vi "ObservedPVs.vi"(8 "error in":errorcluster[](array[cluster]), 10 "Observed PVs":cluster{"PV-Name":string, "n-Channels?":bool}[](array[cluster])=[{"PV-Name"="Waveform", "n-Channels?"=FALSE}, {"PV-Name"="VerticalRange", "n-Channels?"=TRUE}], 11 "PVs":T1(array[cluster])) -> (0 "error out":errorcluster[](array[cluster]), 3 "PVs":T1(array[cluster]))   [LabVIEW 2015, in "CS++ScopeGui.lvlib" / "CS++ScopeGui.lvclass"]
uses:
  CS++ScopeGui.lvclass
  CSPP_Core/Actors/CS++GUIActor Messages/Update-PV Msg/Update-PV Msg.lvclass
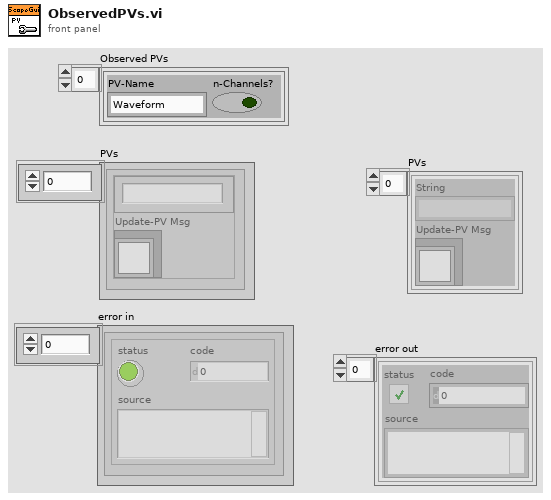
[diagram p1: front panel]
types:
  T1 = cluster{"String":string, "Update-PV Msg":refnum<class "Update-PV Msg.lvclass">}[]
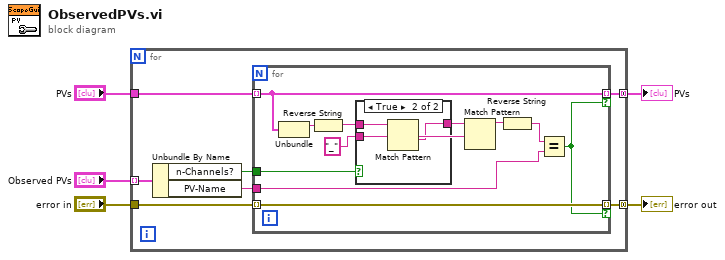
[diagram p0: block diagram]
diagram:
  n1 = for {
    tunnel: "Observed PVs" -> [w12] mode=indexing
    tunnel: "PVs" -> [w11]
    tunnel: "error in" -> [w9]
    tunnel: [w8] -> w3 mode=concatenating
    tunnel: [w10] -> w2 mode=concatenating
    n2 = Unbundle By Name(w12) -> ("n-Channels?"=w7:bool, "PV-Name"=w6:string)
    n3 = for {
      tunnel: w11 -> [w22] mode=indexing
      tunnel: [w22] -> w10 mode=indexing if=w19
      tunnel: w9 -> [w20] mode=indexing
      tunnel: [w20] -> w8 mode=indexing if=w19
      tunnel: w7 -> [w18]
      tunnel: w6 -> [w17]
      w13 = "_" ("regular expression")
      n4 = Unbundle(w22) -> ("String"=w23:string)  [unwired: 1 out]
      n5 = Reverse String(1:w23) -> (0:w16:string)
      n6 = case shown="True" w18 {
        tunnel: w16 -> [w24 w27]
        tunnel: w13 -> [_ w26]
        tunnel: [w24 w25] -> w15
        frame False {
        }
        frame True {
          n7 = Match Pattern(string=w27, regular expression=w26) -> (after substring=w25:string)  [unwired: 1 in, 3 out]
        }
      }
      n8 = Match Pattern(string=w15, regular expression=w13) -> (before substring=w14:string)  [unwired: 1 in, 3 out]
      n9 = Reverse String(1:w14) -> (0:w21:string)
      n10 = Equal?(x=w21, y=w17) -> (x = y?=w19:bool)
    }
  }
  "error out" <- w3
  "PVs" <- w2
